vi "Launch Config Monitor.vi"(8 "error in (no error)":errorcluster, 11 "System Config Module in":refnum<class "System Config Module.lvclass">) -> (0 "error out":errorcluster, 3 "System Config Module out":refnum<class "System Config Module.lvclass">)   [LabVIEW 2020, in "Volatus.lvlib" / "System Config Module.lvclass"]
uses:
  System Config Module.lvclass
  C:/dev/lv20CE/relink/lv-volatus/Volatus/Module/Module.lvclass
  VolatusConfig/VolatusConfigElement/VolatusConfigElement.lvclass
  System Config Module.lvclass/System Config Module.ctl
  Config Alert Module/Config Alert Module.lvclass
  lv-builder/Builder Core/Builder Core.lvlib
  Module/Module.lvclass
  C:/dev/lv20CE/relink/lv-volatus/Volatus/Config Alert Module/Config Alert Module.lvclass
  C:/dev/lv20CE/relink/lv-volatus/Volatus/System Config Server/System Config Module.lvclass
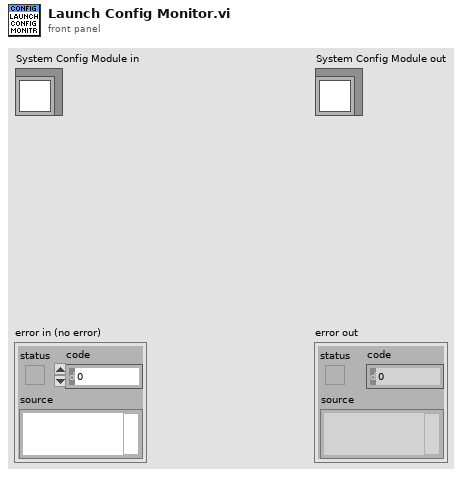
[diagram p1: front panel]
types:
  T1 = typedef "Builder Core.lvlib/Version.ctl" = cluster{"Major":u16, "Minor":u16, "Fix":u16, "Build":u16}
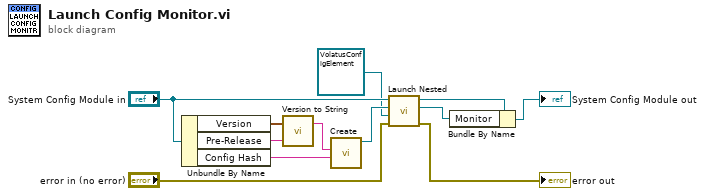
[diagram p0: block diagram]
diagram:
  n1 = Unbundle By Name("System Config Module in") -> ("Version"=w12:T1, "Pre-Release"=w11:string, "Config Hash"=w9:string)
  n2 = call "Version to String.vi"("Version"=w12, "Pre-Release (None)"=w11) -> ("Version String"=w10:string)  [unwired: 5 in]
  n3 = call "Create.vi"("Config Hash"=w9, "Config Version"=w10) -> ("Config Alert Module out"=w6:refnum<class "Config Alert Module.lvclass">)  [unwired: 8 in, 1 out]
  n4 = call "Launch Nested.vi"("error in (no error)"="error in (no error)", "Config Element"=refnum<class "VolatusConfigElement.lvclass"> refnum, "Nested Module"=w6, "Parent in"="System Config Module in") -> ("error out"=→"error out":errorcluster, "MessageQ"=w1:refnum<class "MessageQ.lvclass">, "Parent out"=w7:refnum<class "System Config Module.lvclass">)  [unwired: 5 in]
  n5 = Bundle By Name(cluster=w7, "Monitor"=w1) -> (→"System Config Module out":refnum<class "System Config Module.lvclass">)
